vi "2021 Advent puzzle 04 prepare data.vi"(11 "Bingo boards":string) -> (3 "array type (2D Dbl)":i16[][][](array[numeric]))   [LabVIEW 2021]
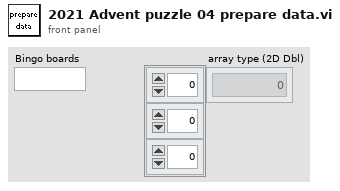
[diagram p1: front panel]
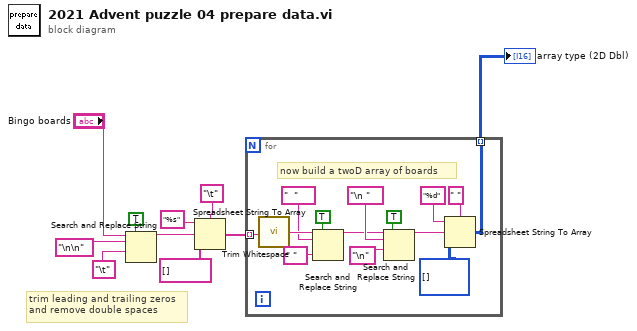
[diagram p0: block diagram]
diagram:
  # "trim leading and trailing zeros\nand remove double spaces"
  n1 = Search and Replace String(replace all?=TRUE ("replace all? (F)"), input string="Bingo boards", search string="\n\n" ("replace string (\"\")"), replace string="\t" ("replace string (\"\")")) -> (result string=w5:string)  [unwired: 4 in, 3 out]
  n2 = Spreadsheet String To Array(delimiter (Tab)="\t", format string="%s", spreadsheet string=w5, array type (2D Dbl)=string[] []) -> (array=w8:string[])
  n3 = for {
    tunnel: [w24] -> w9 mode=indexing
    tunnel: w8 -> [w23] mode=indexing
    # "now build a twoD array of boards"
    n4 = call <vilib>:"Trim Whitespace.vi"("string"=w23) -> ("trimmed string"=w22:string)  [unwired: 1 in]
    n5 = Search and Replace String(replace all?=TRUE ("replace all? (F)"), input string=w22, search string="  " ("replace string (\"\")"), replace string=" " ("replace string (\"\")")) -> (result string=w12:string)  [unwired: 4 in, 3 out]
    n6 = Search and Replace String(replace all?=TRUE ("replace all? (F)"), input string=w12, search string="\n " ("replace string (\"\")"), replace string="\n" ("replace string (\"\")")) -> (result string=w11:string)  [unwired: 4 in, 3 out]
    n7 = Spreadsheet String To Array(delimiter (Tab)=" ", format string="%d", spreadsheet string=w11, array type (2D Dbl)=i16[][] []) -> (array=w24:i16[][])
  }
  "array type (2D Dbl)" <- w9
